vi "Raw Data.vi"(0 "reference in":refnum<class "AD.lvclass">, 5 "error in (no error)":errorcluster) -> (14 "reference out":refnum<class "AD.lvclass">, 15 "Raw Data":dbl, 19 "error out":errorcluster)   [LabVIEW 2013, in "AD.lvclass"]
uses:
  AD.lvclass
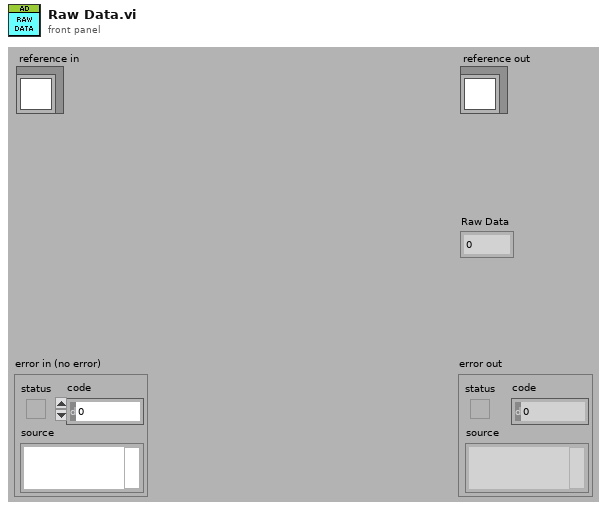
[diagram p1: front panel]
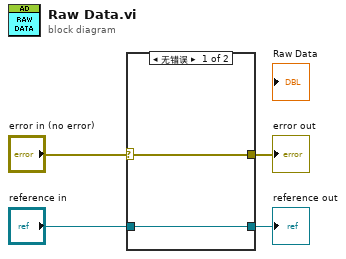
[diagram p0: block diagram]
diagram:
  n1 = case shown="无错误" "error in (no error)" {
    selector: "error in (no error)" -> [w5 w8]
    tunnel: [w5 w8] -> w3
    tunnel: [w6 w7] -> w1
    tunnel: "reference in" -> [w6 w7]
    frame No Error {
    }
    frame Error {
    }
  }
  "error out" <- w3
  "reference out" <- w1
